vi "ADO Connection Set Timeout.vi"(8 "error in (no error)":errorcluster caption="错误输入（无错误）", 10 "ConnectionTimeout":i32, 11 "Database Connection 输入":refnum<class "Database Connection.lvclass"> caption="DNL_LabVIEW Object in") -> (0 "error out":errorcluster caption="错误输出", 3 "Database Connection 输出":refnum<class "Database Connection.lvclass"> caption="DNL_LabVIEW Object out")   [LabVIEW 2011, in "Database Connection.lvclass"]
uses:
  Database Connection.lvclass
  Database Connection.lvclass/Database Connection.ctl
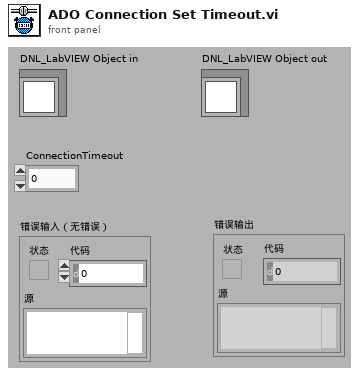
[diagram p1: front panel]
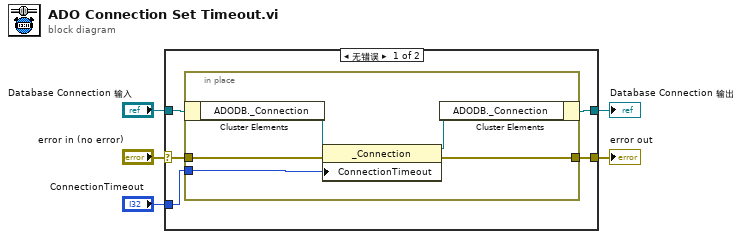
[diagram p0: block diagram]
diagram:
  n1 = case shown="无错误" "error in (no error)" {
    selector: "error in (no error)" -> [w9 w17]
    tunnel: [w8 w17] -> w4
    tunnel: [w6 w16] -> w2
    tunnel: "Database Connection 输入" -> [w10 w16]
    tunnel: "ConnectionTimeout" -> [w7 _]
    frame No Error {
      n2 = in-place {
        in-place-border: w9 -> [w13]
        in-place-border: [w12] -> w8
        in-place-border: w7 -> [w11]
        n3 = in-place-cluster #1(w10) -> ("ADODB._Connection"=w15:refnum<k7>)
        n4 = property class="_Connection"(reference=w15, error in=w13, "ConnectionTimeout"=w11) -> (reference out=w14:refnum<k7>, error out=w12:errorcluster)
        n5 = in-place-cluster #1("ADODB._Connection"=w14) -> (w6:refnum<class "Database Connection.lvclass">)
      }
    }
    frame Error {
    }
  }
  "error out" <- w4
  "Database Connection 输出" <- w2
